vi "Get SMO HELP.vi"(8 "error in (no error)":errorcluster, 10 "Command":string, 11 "Instrument.Oxford1820 in":refnum<class "Instrument.Oxford1820.lvclass">) -> (0 "error out":errorcluster, 2 "help cluster":T1, 3 "Instrument.Oxford1820 out":refnum<class "Instrument.Oxford1820.lvclass">)   [LabVIEW 2019, in "Instrument.Oxford1820.lvclass"]
uses:
  Instrument.Oxford1820.lvclass
  <userlib>/LevyLab/Instrument Framework/subsystems/Help/typedefs/Help--cluster.ctl
  Typedefs/getLN2Level--Cluster.ctl
  Typedefs/getLHeLevel--Cluster.ctl
  <userlib>/LevyLab/Instrument Framework/Instrument Types/Cryostat/Typedefs/Magnet Axis--Enum.ctl
  <userlib>/LevyLab/Instrument Framework/Instrument Types/Cryostat/Typedefs/getMagnet--cluster.ctl
  <userlib>/LevyLab/Instrument Framework/Instrument Types/Cryostat/Typedefs/setMagnet--cluster.ctl
  <userlib>/LevyLab/Instrument Framework/Instrument Types/Cryostat/Typedefs/Magnet Mode--Enum.ctl
  <userlib>/LevyLab/Instrument Framework/Instrument Types/Cryostat/Instrument.Cryostat.lvclass
  <userlib>/LevyLab/Instrument Framework/subsystems/Help/Help.lvclass
  <userlib>/LevyLab/Instrument Framework/Instrument/Typedefs/Instrument.Commands--Enum.ctl
  <userlib>/LevyLab/Instrument Framework/Instrument/Instrument.lvclass
  <userlib>/LevyLab/Instrument Framework/Instrument/Typedefs/Instrument.IDN--cluster.ctl
  <vilib>/PRIrvin/JSON-Schema/JSON-Schema.lvlib
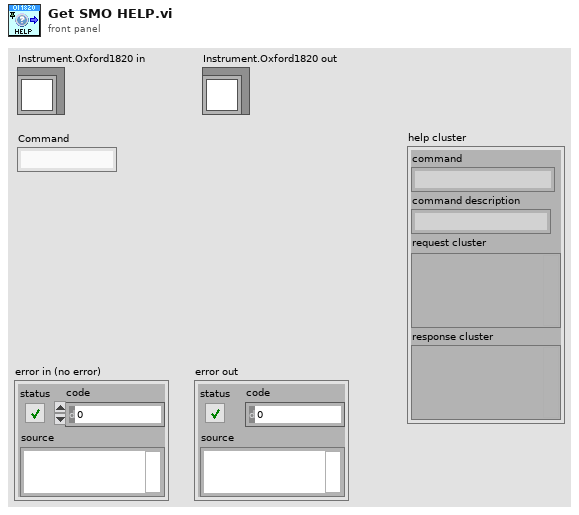
[diagram p1: front panel]
types:
  T1 = typedef "Instrument.lvlib/Help.lvclass/Help--cluster.ctl" = cluster{"command":string, "command description":string, "request cluster":variant, "response cluster":variant}
  T2 = typedef "Instrument.Oxford1820.lvclass/getLN2Level--Cluster.ctl" = cluster{"LN2Level":dbl}
  T3 = typedef "Instrument.Oxford1820.lvclass/getLHeLevel--Cluster.ctl" = cluster{"LHeLevel":dbl}
  T4 = typedef "Instrument.Cryostat.lvclass/getMagnet--cluster.ctl" = cluster{"field":dbl, "status":string, "finished":bool}
  T5 = typedef "Instrument.Cryostat.lvclass/Magnet Axis--Enum.ctl" = enum16{"X", "Y", "Z"}
  T6 = typedef "Instrument.Cryostat.lvclass/setMagnet--cluster.ctl" = cluster{"field":dbl, "rate":dbl, "axis":T5, "mode":T7}
  T7 = typedef "Instrument.Cryostat.lvclass/Magnet Mode--Enum.ctl" = enum16{"Persistent", "Driven"}
  T8 = typedef "Instrument.lvlib/Instrument.lvclass/Instrument.Commands--Enum.ctl" = enum16{"ACK", "HELP", "IDN", "getAll", "getAllData"}
  T9 = typedef "Instrument.lvlib/Instrument.lvclass/Instrument.IDN--cluster.ctl" = cluster{"vendor":string, "model":string, "serial":string, "firmware":string}
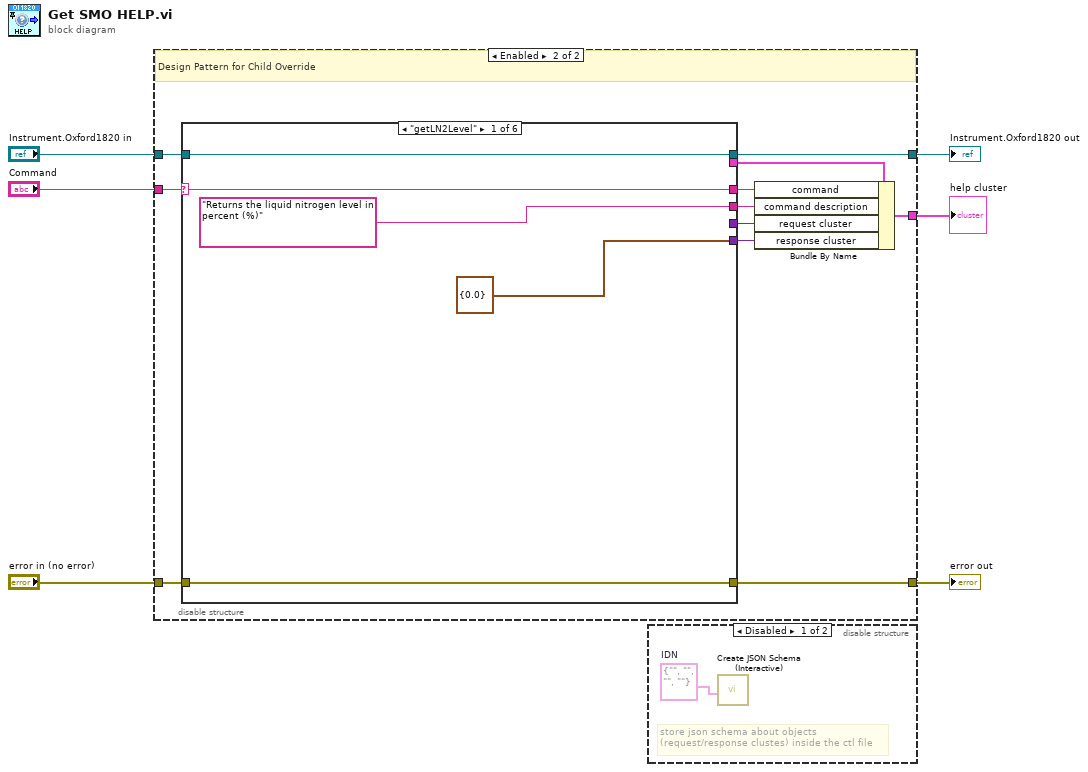
[diagram p0: block diagram]
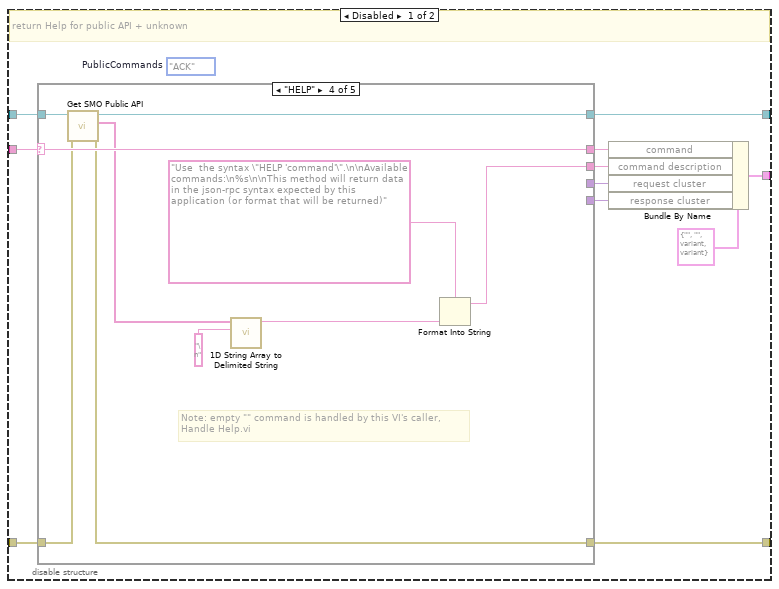
[diagram p3: hidden frame]
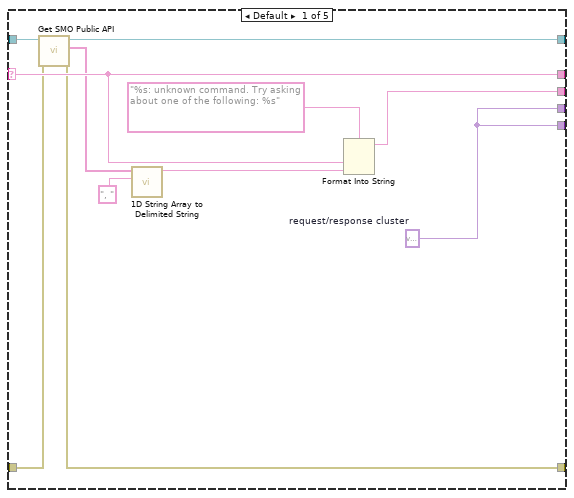
[diagram p4: hidden frame]
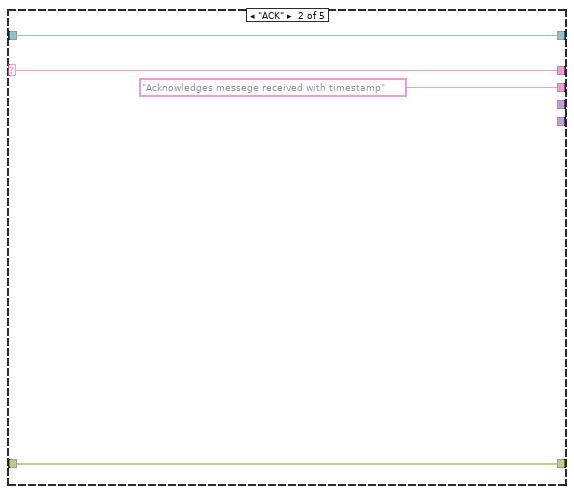
[diagram p5: hidden frame]
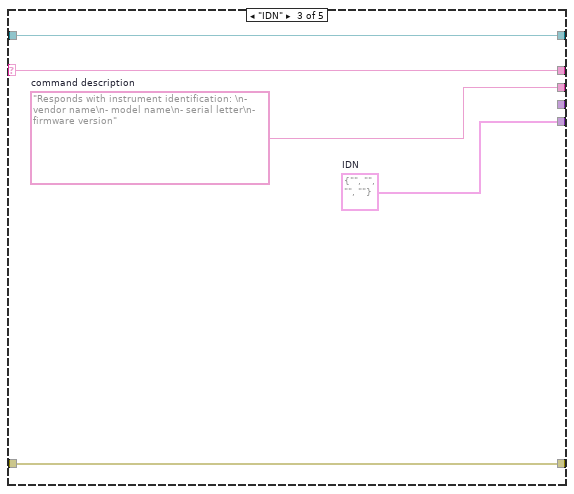
[diagram p6: hidden frame]
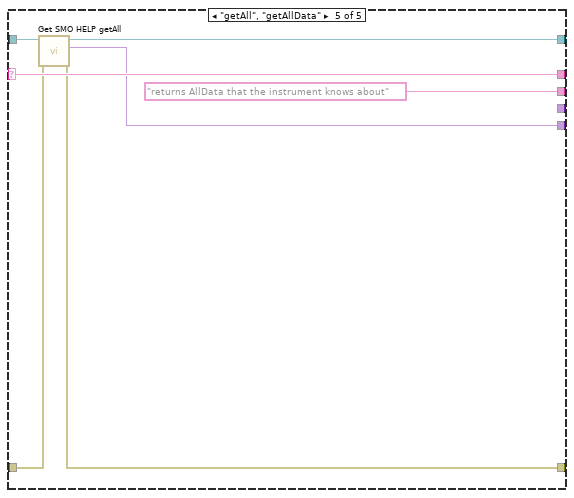
[diagram p7: hidden frame]
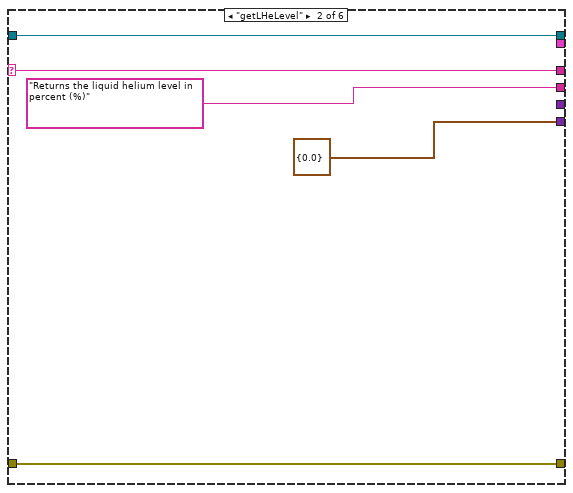
[diagram p8: hidden frame]
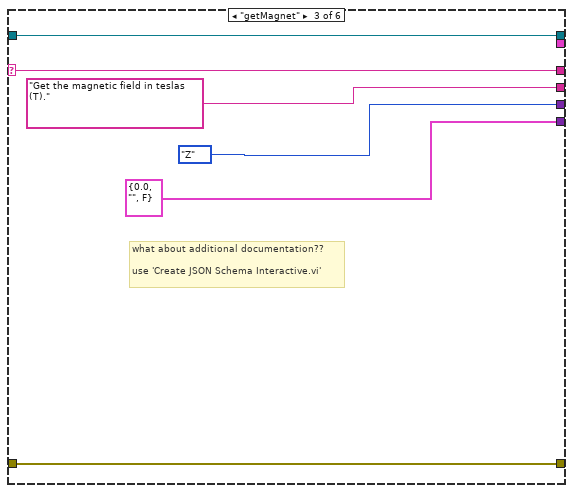
[diagram p9: hidden frame]
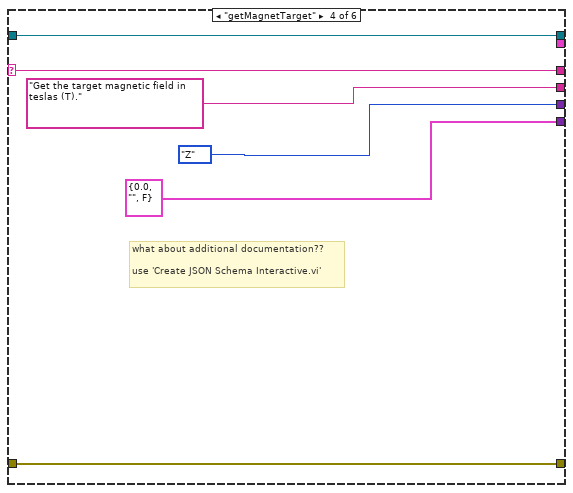
[diagram p10: hidden frame]
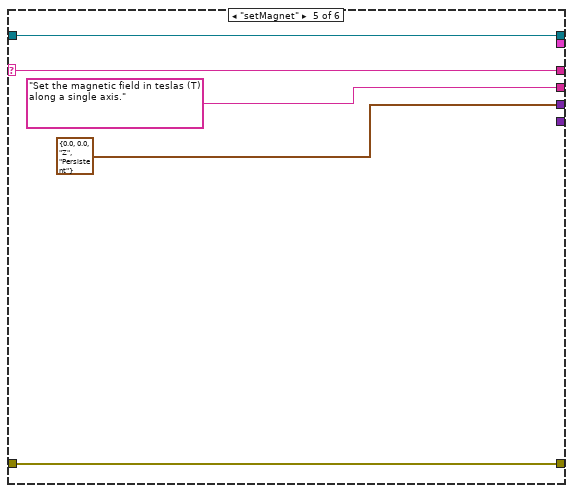
[diagram p11: hidden frame]
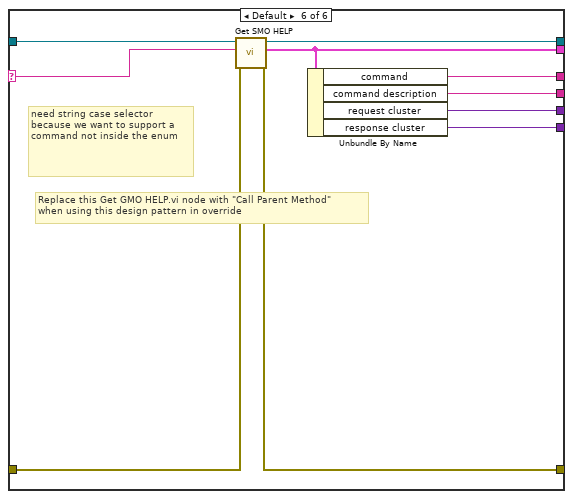
[diagram p12: hidden frame]
diagram:
  n1 = disable-structure shown="Enabled" {
    disable-tunnel: [w17 w57] -> w4
    disable-tunnel: "Instrument.Oxford1820 in" -> [w16 w58]
    disable-tunnel: "error in (no error)" -> [w15 w63]
    disable-tunnel: [w11 w65] -> w6
    disable-tunnel: [w8 w64] -> w5
    disable-tunnel: "Command" -> [w7 w55]
    frame Disabled {
      (unwired) Instrument.Commands--Enum."ACK"  # PublicCommands
      # "return Help for public API + unknown"
      n2 = case shown="\"HELP\"" w7 {
        selector: w7 -> [w24 w30 w36 w44 w53]
        tunnel: w15 -> [w21 w32 w34 w41 w52]
        tunnel: [w22 w32 w34 w42 w51] -> w11
        tunnel: [w26 "Acknowledges messege received with timestamp" w37 w38 "returns AllData that the instrument knows about"] -> w13
        tunnel: [w19 _ _ _ _] -> w12
        tunnel: [w19 _ w33 _ w48] -> w10
        tunnel: [w24 w30 w36 w44 w53] -> w14
        tunnel: w16 -> [w23 w29 w35 w43 w49]
        tunnel: [w20 w29 w35 w40 w50] -> w17
        frame Default {
          w19 = variant  # request/response cluster
          n3 = call-dynamic "Get SMO Public API.vi"("error in (no error)"=w21, "Instrument.Example In"=w23) -> ("error out"=w22:errorcluster, "Commands"=w18:string[], "Instrument.Example out"=w20:refnum<class "Instrument.Oxford1820.lvclass">)  [unwired: 7 in]
          n4 = call <vilib>:"1D String Array to Delimited String.vi"("delimiter"=", ", "string array"=w18) -> ("delimited string"=w27:string)  [unwired: 9 in]
          n5 = Format Into String(format string="%s: unknown command. Try asking about one of the following: %s", w24, w27) -> (resulting string=w26:string)  [unwired: 2 in, 1 out]
        }
        frame "ACK" {
        }
        frame "IDN" {
          w33 = T9 {"vendor"="", "model"="", "serial"="", "firmware"=""}  # IDN
          w37 = "Responds with instrument identification: \n- vendor name\n- model name\n- serial letter\n- firmware version"  # command description
        }
        frame "HELP" {
          # "Note: empty \"\" command is handled by this VI's caller,\nHandle Help.vi"
          n6 = call-dynamic "Get SMO Public API.vi"("error in (no error)"=w41, "Instrument.Example In"=w43) -> ("error out"=w42:errorcluster, "Commands"=w39:string[], "Instrument.Example out"=w40:refnum<class "Instrument.Oxford1820.lvclass">)  [unwired: 7 in]
          n7 = call <vilib>:"1D String Array to Delimited String.vi"("delimiter"="\n", "string array"=w39) -> ("delimited string"=w47:string)  [unwired: 9 in]
          n8 = Format Into String(format string="Use  the syntax \"HELP 'command'\".\n\nAvailable commands:\n%s\n\nThis method will return data in the json-rpc syntax expected by this application (or format that will be returned)", w47) -> (resulting string=w38:string)  [unwired: 2 in, 1 out]
        }
        frame "getAll", "getAllData" {
          n9 = call-dynamic "Get SMO HELP getAll.vi"("error in (no error)"=w52, "Instrument in"=w49) -> ("error out"=w51:errorcluster, "getAll response cluster"=w48:variant, "Instrument out"=w50:refnum<class "Instrument.Oxford1820.lvclass">)  [unwired: 7 in]
        }
      }
      n10 = Bundle By Name(cluster=T1 {"command"="", "command description"="", "request cluster"=variant, "response cluster"=variant} ("Help"), "command"=w14, "command description"=w13, "request cluster"=w12, "response cluster"=w10) -> (w8:T1)
    }
    frame Enabled {
      # "Design Pattern for Child Override"
      n11 = case shown="\"getLN2Level\"" w55 {
        selector: w55 -> [w70 w75 w81 w87 w92 w101]
        tunnel: [w70 w75 w81 w87 w92 w96] -> w62
        tunnel: w63 -> [w69 w74 w80 w86 w91 w94]
        tunnel: [w69 w74 w80 w86 w91 w93] -> w65
        tunnel: ["Returns the liquid nitrogen level in percent (%)" "Returns the liquid helium level in percent (%)" "Get the magnetic field in teslas (T)." "Get the target magnetic field in teslas (T)." "Set the magnetic field in teslas (T) along a single axis." w97] -> w61
        tunnel: [_ _ Magnet_Axis--Enum."Z" ("Axis") Magnet_Axis--Enum."Z" ("Axis") T6 {"field"=0.0, "rate"=0.0, "axis"=enum."Z", "mode"=enum."Persistent"} ("Set Magnet Field") w98] -> w60
        tunnel: [T2 {"LN2Level"=0.0} ("getN2Level") T3 {"LHeLevel"=0.0} ("getHeLevel") T4 {"field"=0.0, "status"="", "finished"=FALSE} ("getMagnet") T4 {"field"=0.0, "status"="", "finished"=FALSE} ("getMagnet") _ w99] -> w59
        tunnel: w58 -> [w67 w72 w78 w84 w89 w102]
        tunnel: [w67 w72 w78 w84 w89 w100] -> w57
        tunnel: [_ _ _ _ _ w95] -> w56
        frame "getLN2Level" {
        }
        frame "getLHeLevel" {
        }
        frame "getMagnet" {
          # "what about additional documentation??\n\nuse 'Create JSON Schema Interactive.vi'"
        }
        frame "getMagnetTarget" {
          # "what about additional documentation??\n\nuse 'Create JSON Schema Interactive.vi'"
        }
        frame "setMagnet" {
        }
        frame Default {
          # "need string case selector because we want to support a command not inside the enum"
          # "Replace this Get GMO HELP.vi node with \"Call Parent Method\"\nwhen using this design pattern in override"
          n12 = call-parent "Get SMO HELP.vi"("error in (no error)"=w94, "Command"=w101, "Instrument.Cryostat in"=w102) -> ("error out"=w93:errorcluster, "help cluster"=w95:T1, "Instrument.Cryostat out"=w100:refnum<class "Instrument.Oxford1820.lvclass">)  [unwired: 6 in]
          n13 = Unbundle By Name(w95) -> ("command"=w96:string, "command description"=w97:string, "request cluster"=w98:variant, "response cluster"=w99:variant)
        }
      }
      n14 = Bundle By Name(cluster=w56, "command"=w62, "command description"=w61, "request cluster"=w60, "response cluster"=w59) -> (w64:T1)
    }
  }
  "Instrument.Oxford1820 out" <- w4
  "help cluster" <- w5
  "error out" <- w6
  n15 = disable-structure shown="Disabled" {
    frame Disabled {
      w103 = T9 {"vendor"="", "model"="", "serial"="", "firmware"=""}  # IDN
      # "store json schema about objects\n(request/response clustes) inside the ctl file"
      n16 = call <vilib>:"Create JSON Schema (Interactive).vi"("LV Object"=w103) -> ()  [unwired: 9 in, 2 out]
    }
    frame Enabled {
    }
  }
